vi "try_Show Hidden Controls While Editing.vi"() -> ()   [LabVIEW 2025]
panel:
  in  "Hide B&C":bool
  in  "Button 2":bool
  in  "Button":bool
  in  "Chose a day":i32(listbox)
  out "File Path out":path
  out "Boolean out":bool
  out "String out":string
  out "Numeric out":dbl
  in  "File Path in":path
  in  "Boolean in":bool
  in  "String in":string
  in  "Numeric in":dbl
  # "Scenario\nSee hidden controls on the front panel at edit time.\n\nInstructions\n1. In edit mode right click any of the controls or indicator and then Advanced>>Hide Control\n2. Alternatively Run the VI and click HIDE ALL CONTROLS AND INDICATORS to hide all the controls and indicators \n3. To show the Hidden controls in edit mode select Edit > Show Hidden Controls While Editing"
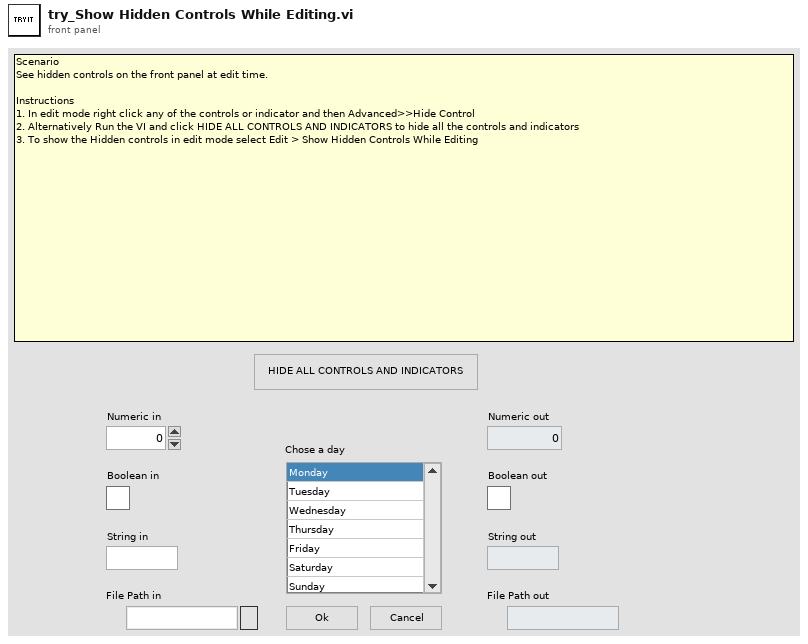
[diagram p1: front panel]
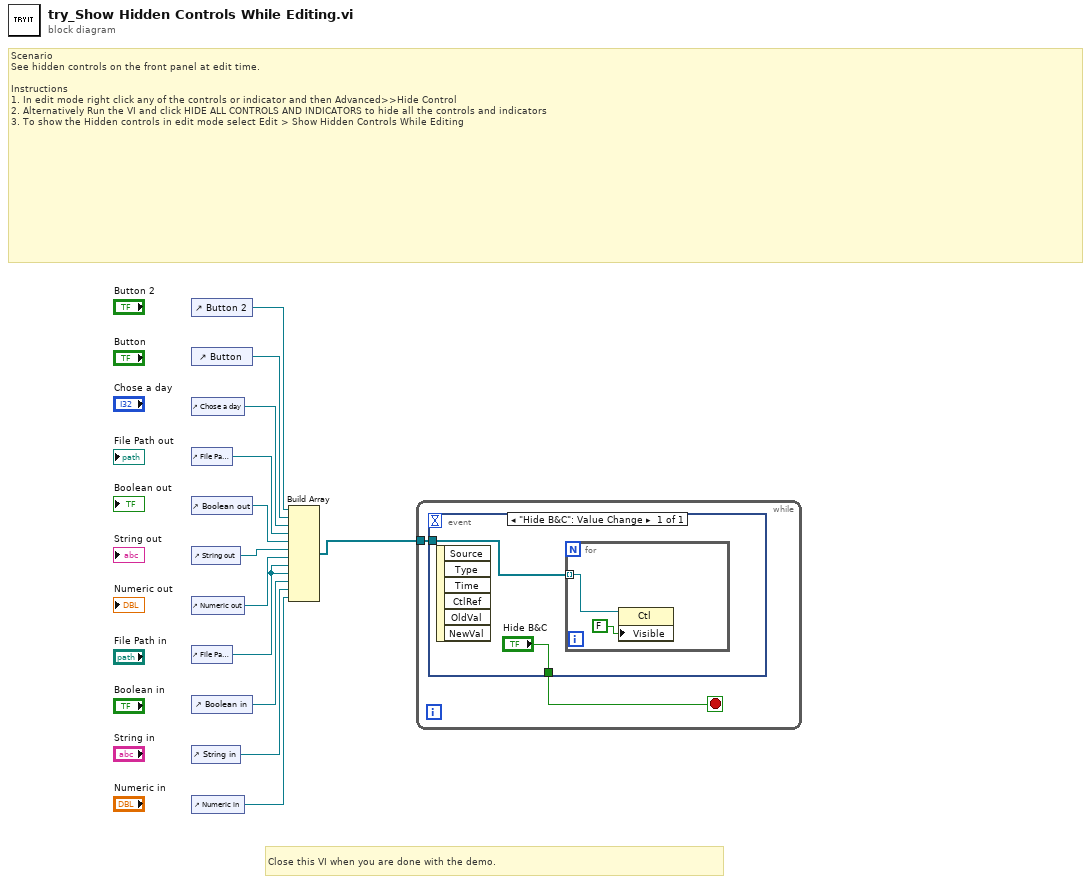
[diagram p0: block diagram]
diagram:
  # "Close this VI when you are done with the demo."
  # "Scenario\nSee hidden controls on the front panel at edit time.\n\nInstructions\n1. In edit mode right click any of the controls or indicator and then Advanced>>Hide Control\n2. Alternatively Run the VI and click HIDE ALL CONTROLS AND INDICATORS to hide all the controls and indicators \n3. To show the Hidden controls in edit mode select Edit > Show Hidden Controls While Editing"
  n1 = control-ref of="Button 2"() -> (w12:refnum<vi>)
  n2 = control-ref of="Button"() -> (w11:refnum<vi>)
  n3 = control-ref of="Chose a day"() -> (w10:refnum<vi>)
  n4 = control-ref of="File Path out"() -> (w9:refnum<vi>)
  n5 = control-ref of="Boolean out"() -> (w8:refnum<vi>)
  n6 = control-ref of="String out"() -> (w7:refnum<vi>)
  n7 = control-ref of="Numeric out"() -> (w6:refnum<vi>)
  n8 = control-ref of="File Path in"() -> (w5:refnum<vi>)
  n9 = control-ref of="Boolean in"() -> (w4:refnum<vi>)
  n10 = control-ref of="String in"() -> (w3:refnum<vi>)
  n11 = control-ref of="Numeric in"() -> (w2:refnum<vi>)
  n12 = Build Array(w12, w11, w10, w9, w8, w7, w6, w5, w5, w4, w3, w2) -> (w1:refnum<vi>[])
  n13 = while {
    tunnel: w1 -> [w13]
    stop <- w14 stop-if-true
    n14 = event shown="[0] \"Hide B&C\": Value Change" {
      selector: _ -> [_]
      dyn-events: _ -> [_]
      timeout: _ -> [_]
      tunnel: ["Hide B&C"] -> w14
      tunnel: w13 -> [w15]
      event "Hide B&C": Value Change {
        n15 = event-data() -> ()  [unwired: 1 in, 6 out]
        n16 = for {
          tunnel: w15 -> [w17] mode=indexing
          n17 = property class="Ctl"(reference=w17, "Visible"=FALSE) -> ()  [unwired: 1 in, 2 out]
        }
      }
    }
  }
